vi "module config version constant.vi"() -> (3 "version":string="1.0.0.0")   [LabVIEW 2013, in "TBM module configuration.lvclass"]
uses:
  TBM module configuration.lvclass
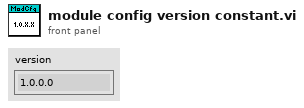
[diagram p1: front panel]
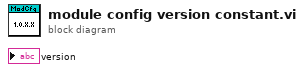
[diagram p0: block diagram]
diagram:
